vi "readForceSensor.vi"(8 "error in (no error)":errorcluster, 11 "Model in":refnum<class "Model.lvclass">) -> (0 "error out":errorcluster, 3 "Model out":refnum<class "Model.lvclass">)   [LabVIEW 2015, in "Model.lvclass"]
uses:
  Model.lvclass
  <userlib>/Common/Devices/ForceSensorCalculator/ForceSensorCalculator/ForceSensorCalculator.lvclass
  ILCADCFactory/ILCADCFactory/ILCADCFactory.lvclass
  Model.lvclass/Model.ctl
  <userlib>/Common/Devices/ForceSensorCalculator/ForceSensorCalculator/ForceSensorCalculator.lvclass/ForceSensorCalculator.ctl
  ILCADC/IILCADC/IILCADC.lvclass
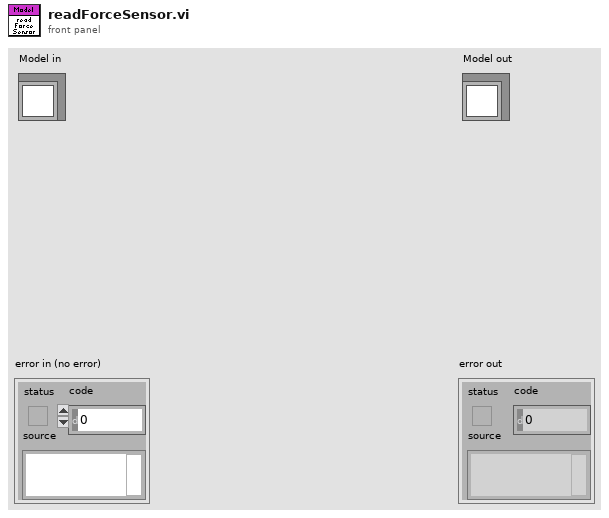
[diagram p1: front panel]
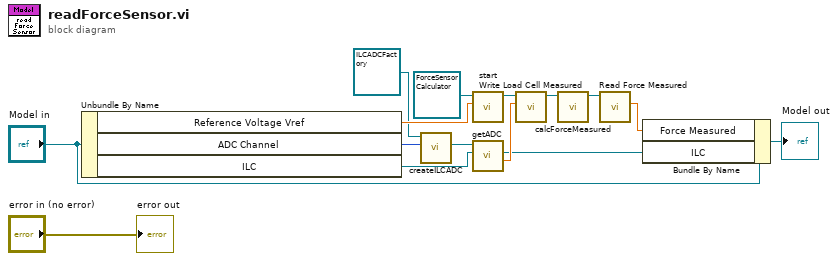
[diagram p0: block diagram]
diagram:
  n1 = Unbundle By Name("Model in") -> ("Reference Voltage Vref"=w14:dbl[unit], "ADC Channel"=w12:u8, "ILC"=w10:refnum<class "ILC.lvclass">)
  n2 = call-dynamic "createILCADC.vi"("Channel"=w12, "ILCADCFactory in"=refnum<class "ILCADCFactory.lvclass"> refnum) -> ("ILCADC"=w11:refnum<class "IILCADC.lvclass">)  [unwired: 7 in, 2 out]
  n3 = call <userlib>:"start.vi"("Reference Voltage Vref"=w14, "ForceSensor in"=refnum<class "ForceSensorCalculator.lvclass"> refnum) -> ("ForceSensor out"=w13:refnum<class "ForceSensorCalculator.lvclass">)  [unwired: 8 in, 1 out]
  n4 = call-dynamic "getADC.vi"("ILC In"=w10, "IILCADC in"=w11) -> ("ADC Value"=w9:dbl[unit], "ILC Out"=w6:refnum<class "ILC.lvclass">)  [unwired: 6 in, 2 out]
  n5 = call <userlib>:"Write Load Cell Measured.vi"("Load Cell Measured"=w9, "ForceSensor in"=w13) -> ("ForceSensor out"=w8:refnum<class "ForceSensorCalculator.lvclass">)  [unwired: 9 in]
  n6 = call <userlib>:"calcForceMeasured.vi"("ForceSensor in"=w8) -> ("ForceSensor out"=w7:refnum<class "ForceSensorCalculator.lvclass">)  [unwired: 9 in, 1 out]
  n7 = call <userlib>:"Read Force Measured.vi"("ForceSensor in"=w7) -> ("Force Demand"=w3:dbl[unit])  [unwired: 9 in, 1 out]
  n8 = Bundle By Name(cluster="Model in", "Force Measured"=w3, "ILC"=w6) -> (→"Model out":refnum<class "Model.lvclass">)
  "error out" <- "error in (no error)"
